vi "Swap Mutation.vi"(8 "error in (no error)":errorcluster, 11 "GA in":refnum<class "GA.lvclass">) -> (0 "error out":errorcluster, 3 "GA out":refnum<class "GA.lvclass">)   [LabVIEW 2013, in "GA.lvclass"]
uses:
  GA.lvclass
  GA.lvclass/GA.ctl
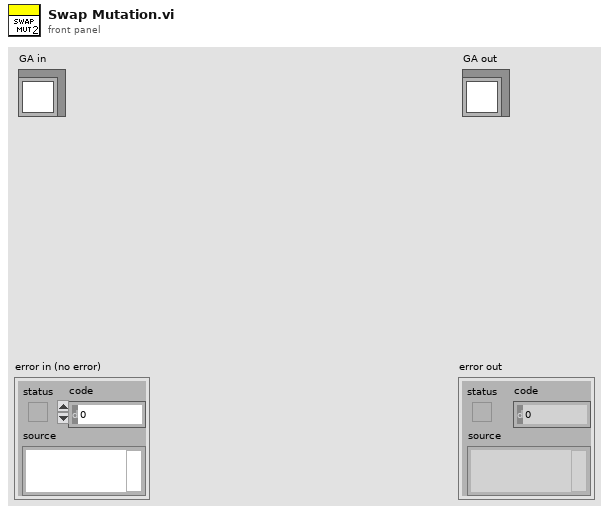
[diagram p1: front panel]
types:
  T1 = typedef "Solution.ctl" = cluster{"Schedule":u16[], "Fitness":u16, "Fitness Valid?":bool}
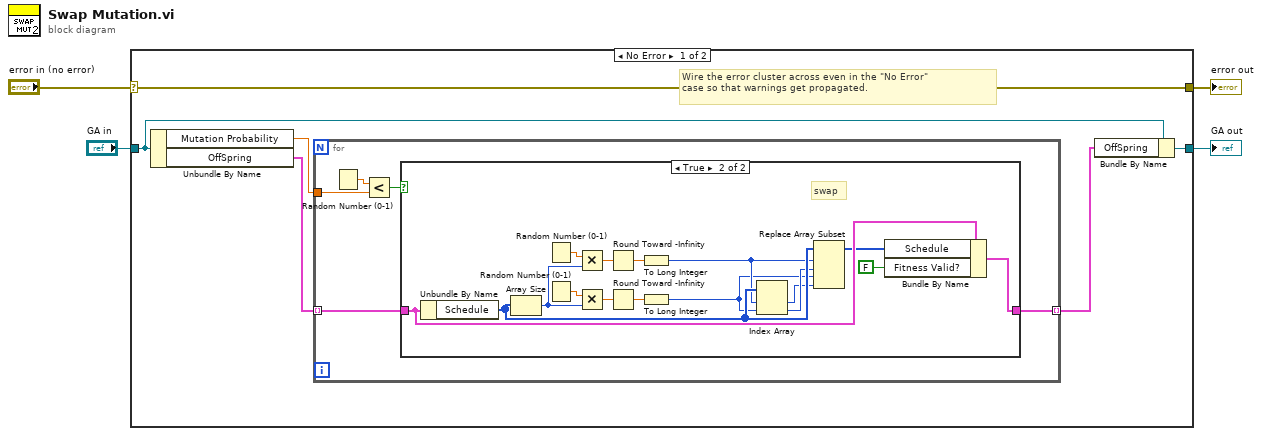
[diagram p0: block diagram]
diagram:
  n1 = case shown="No Error" "error in (no error)" {
    selector: "error in (no error)" -> [w10 w34]
    tunnel: [w10 w34] -> w3
    tunnel: [w5 w33] -> w1
    tunnel: "GA in" -> [w6 w33]
    frame No Error {
      # "Wire the error cluster across even in the \"No Error\"\ncase so that warnings get propagated."
      n2 = Unbundle By Name(w6) -> ("Mutation Probability"=w8:dbl, "OffSpring"=w9:T1[])
      n3 = for {
        tunnel: w9 -> [w13] mode=indexing
        tunnel: w8 -> [w14]
        tunnel: [w11] -> w7 mode=indexing
        n4 = Random Number (0-1)() -> (number: 0 to 1=w15:dbl)
        n5 = Less?(x=w15, y=w14) -> (x < y?=w12:bool)
        n6 = case shown="True" w12 {
          tunnel: w13 -> [w16 w20]
          tunnel: [w16 w17] -> w11
          frame False {
          }
          frame True {
            # "swap"
            n7 = Unbundle By Name(w20) -> ("Schedule"=w27:u16[])
            n8 = Array Size(array=w27) -> (size(s)=w30:i32)
            n9 = Random Number (0-1)() -> (number: 0 to 1=w32:dbl)
            n10 = Random Number (0-1)() -> (number: 0 to 1=w31:dbl)
            n11 = Multiply(x=w32, y=w30) -> (x*y=w29:dbl)
            n12 = Multiply(x=w31, y=w30) -> (x*y=w28:dbl)
            n13 = Round Toward -Infinity(1:w29) -> (0:w26:dbl)
            n14 = Round Toward -Infinity(1:w28) -> (0:w25:dbl)
            n15 = To Long Integer(number=w26) -> (32bit integer=w24:i32)
            n16 = To Long Integer(number=w25) -> (32bit integer=w22:i32)
            n17 = Index Array(array=w27, index #1=w24, index #2=w22) -> (element #1=w21:u16, element #2=w23:u16)
            n18 = Replace Array Subset(array=w27, new element #1=w23, index #1=w24, new element #2=w21, index #2=w22) -> (w19:u16[])
            n19 = Bundle By Name(cluster=w20, "Schedule"=w19, "Fitness Valid?"=FALSE) -> (w17:T1)
          }
        }
      }
      n20 = Bundle By Name(cluster=w6, "OffSpring"=w7) -> (w5:refnum<class "GA.lvclass">)
    }
    frame Error {
    }
  }
  "error out" <- w3
  "GA out" <- w1
